vi "CPF.vi"(1 "CPF Choice":enum32{"CPF Fast", "CPF Accurate"}(radio)=enum."CPF Accurate" caption="CPF Choice  (CPF Accurate)", 2 "y":dbl=1.0, 3 "x":dbl=1.0) -> (0 "CPF":cdb=0.30474420525691254+0.20821893820283166i caption="CPF Value" format="%#_17g")   [LabVIEW 2015]
panel:
  # "Output Section"
  # "Input Section"
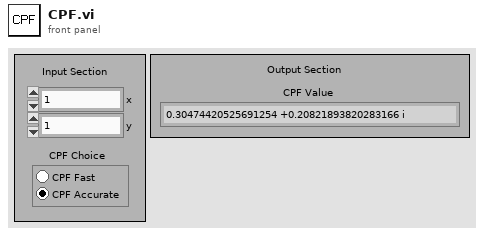
[diagram p1: front panel]
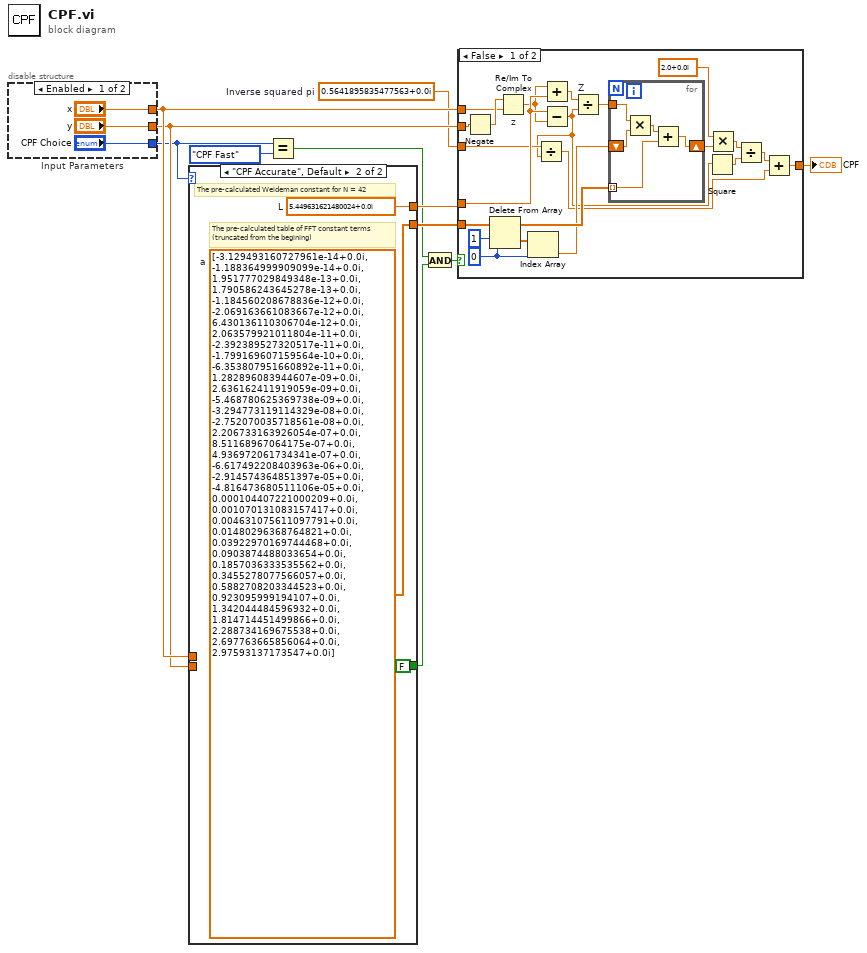
[diagram p0: block diagram]
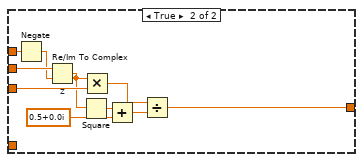
[diagram p2: hidden frame]
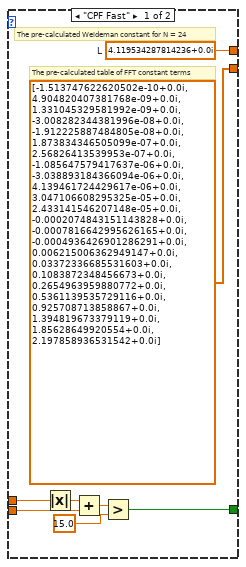
[diagram p3: hidden frame]
diagram:
  w3 = cdb 0.5641895835477563+0.0i  # Inverse squared pi
  n1 = disable-structure "Input Parameters" shown="Enabled" {
    disable-tunnel: ["x" _] -> w8
    disable-tunnel: ["y" _] -> w7
    disable-tunnel: ["CPF Choice" _] -> w2
    frame Enabled {
    }
    frame Disabled {
    }
  }
  n2 = case shown="\"CPF Accurate\", Default" w2 {
    tunnel: [w22 w24] -> w11
    tunnel: [cdb[] [-1.513747622620502e-10+0.0i, 4.904820407381768e-09+0.0i, 1.331045329581992e-09+0.0i, -3.008282344381996e-08+0.0i, -1.912225887484805e-08+0.0i, 1.873834346505099e-07+0.0i, 2.56826413539953e-07+0.0i, -1.085647579417637e-06+0.0i, -3.038893184366094e-06+0.0i, 4.139461724429617e-06+0.0i, 3.047106608295325e-05+0.0i, 2.433141546207148e-05+0.0i, -0.0002074843151143828+0.0i, -0.0007816642995626165+0.0i, -0.0004936426901286291+0.0i, 0.006215006362949147+0.0i, 0.03372336685531603+0.0i, 0.1083872348456673+0.0i, 0.2654963959880772+0.0i, 0.5361139535729116+0.0i, 0.925708713858867+0.0i, 1.394819673379119+0.0i, 1.85628649920554+0.0i, 2.197858936531542+0.0i] ("output array") w25] -> w10
    tunnel: w8 -> [w20 _]
    tunnel: w7 -> [w18 _]
    tunnel: [w15 FALSE] -> w6
    frame "CPF Fast" {
      w22 = cdb 4.119534287814236+0.0i  # L
      # "The pre-calculated Weideman constant for N = 24"
      # "The pre-calculated table of FFT constant terms"
      n3 = Absolute Value(x=w20) -> (abs(x)=w19:dbl)
      n4 = Add(x=w19, y=w18) -> (x+y=w17:dbl)
      n5 = Greater?(x=w17, y=15.0) -> (0:w15:bool)
    }
    frame "CPF Accurate", Default {
      w24 = cdb 5.449631621480024+0.0i  # L
      w25 = cdb[] [-3.129493160727961e-14+0.0i, -1.188364999909099e-14+0.0i, 1.951777029849348e-13+0.0i, 1.790586243645278e-13+0.0i, -1.184560208678836e-12+0.0i, -2.069163661083667e-12+0.0i, 6.430136110306704e-12+0.0i, 2.063579921011804e-11+0.0i, -2.392389527320517e-11+0.0i, -1.799169607159564e-10+0.0i, -6.353807951660892e-11+0.0i, 1.282896083944607e-09+0.0i, 2.636162411919059e-09+0.0i, -5.468780625369738e-09+0.0i, -3.294773119114329e-08+0.0i, -2.752070035718561e-08+0.0i, 2.206733163926054e-07+0.0i, 8.51168967064175e-07+0.0i, 4.936972061734341e-07+0.0i, -6.617492208403963e-06+0.0i, -2.914574364851397e-05+0.0i, -4.816473680511106e-05+0.0i, 0.000104407221000209+0.0i, 0.001070131083157417+0.0i, 0.004631075611097791+0.0i, 0.01480296368764821+0.0i, 0.03922970169744468+0.0i, 0.0903874488033654+0.0i, 0.1857036333535562+0.0i, 0.3455278077566057+0.0i, 0.5882708203344523+0.0i, 0.923095999194107+0.0i, 1.342044484596932+0.0i, 1.814714451499866+0.0i, 2.288734169675538+0.0i, 2.697763665856064+0.0i, 2.97593137173547+0.0i]  # a
      # "The pre-calculated Weideman constant for N = 42"
      # "The pre-calculated table of FFT constant terms\n(truncated from the begining)"
    }
  }
  n6 = Equal?(x=w2, y=enum32{"CPF Fast", "CPF Accurate"}."CPF Fast" ("CPF Choice")) -> (x = y?=w5:bool)
  n7 = And(x=w5, y=w6) -> (x .and. y?=w4:bool)
  n8 = case shown="False" w4 {
    tunnel: w11 -> [w47 _]
    tunnel: w10 -> [w38 _]
    tunnel: [w34 w53] -> w9
    tunnel: w8 -> [w33 w62]
    tunnel: w7 -> [w32 w61]
    tunnel: w3 -> [w31 w59]
    frame False {
      w30 = 0 ("index")
      n9 = Negate(x=w32) -> (-x=w44:dbl)
      n10 = Delete From Array(array=w38, length=1, index=w30) -> (deleted portion=w40:cdb[], array with subset deleted=w41:cdb[])
      n11 = Re/Im To Complex "z"(1:w33, 2:w44) -> (0:w46:cdb)
      n12 = Index Array(array=w40, index=w30) -> (element=w39:cdb)
      n13 = Add(x=w46, y=w47) -> (x+y=w45:cdb)
      n14 = Subtract(x=w47, y=w46) -> (x-y=w26:cdb)
      n15 = Divide(x=w31, y=w26) -> (x/y=w28:cdb)
      n16 = Divide "Z"(x=w45, y=w26) -> (x/y=w43:cdb)
      n17 = for "Output = p" {
        shift-right: [w48] -> w37
        shift-left: w39 -> [w52]
        tunnel: w43 -> [w51]
        tunnel: w41 -> [w49] mode=indexing
        n18 = Multiply(x=w51, y=w52) -> (x*y=w50:cdb)
        n19 = Add(x=w50, y=w49) -> (x+y=w48:cdb)
      }
      n20 = Square(x=w26) -> (x^2=w35:cdb)
      n21 = Multiply(x=cdb 2.0+0.0i, y=w37) -> (x*y=w36:cdb)
      n22 = Divide(x=w36, y=w35) -> (x/y=w27:cdb)
      n23 = Add(x=w27, y=w28) -> (x+y=w34:cdb)
    }
    frame True {
      n24 = Negate(x=w62) -> (-x=w60:dbl)
      n25 = Re/Im To Complex "z"(1:w60, 2:w61) -> (0:w58:cdb)
      n26 = Square(x=w58) -> (x^2=w57:cdb)
      n27 = Multiply(x=w58, y=w59) -> (x*y=w54:cdb)
      n28 = Add(x=w57, y=cdb 0.5+0.0i) -> (x+y=w55:cdb)
      n29 = Divide(x=w54, y=w55) -> (x/y=w53:cdb)
    }
  }
  "CPF" <- w9
